vi "Math - Compute Impulse Response.vi"(0 "reference in":refnum<class "GSwFormDSP.lvclass">, 5 "error in (no error)":errorcluster) -> (14 "reference out":refnum<class "GSwFormDSP.lvclass">, 19 "error out":errorcluster)   [LabVIEW 2020, in "GSwFormDSP.lvclass"]
uses:
  GSwFormDSP.lvclass
  Attribute List.ctl
  Attribute Options.ctl
  <vilib>/Analysis/2dsp.llb/Inverse Real FFT.vi
  <vilib>/Analysis/NI_AALPro.lvlib
panel:
  out "Fs":dbl
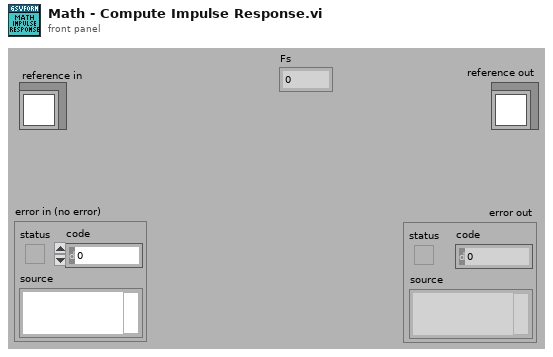
[diagram p1: front panel]
types:
  T1 = typedef "GSwFormDSP.lvclass/Attribute Options.ctl" = enum16{"Append to Attribute using \"( )\"", "Replace Attribute Value"}
  T2 = typedef "GSwFormDSP.lvclass/Attribute List.ctl" = string
  T3 = typedef "GSwFormDSP.lvclass/ObjectAttributes.ctl" = cluster{"Wform Ref":refnum<data-value>, "Nb Signals":i32, "Spectral Function Parameters":T4, "FFT":waveform(cdb)[], "Nb FFT":i32, "Nb Averages":i32[], "Reference Indexes":i32[], "Response Indexes":i32[], "Coherence":waveform(dbl)[], "TDF Parameters":T6, "DAQ":cluster{"Duration (sec)":dbl, "Buffer Size (Samples)":i32, "Offset (Samples)":i32}, "Filter Impulse Response (TDF)":waveform(dbl), "Sound Playback":T7}
  T4 = typedef "GSwFormDSP.lvclass/Spectral Parameters.ctl" = cluster{"Frequency resolution (Hz)":dbl, "Overlap":dbl, "Window":T5}
  T5 = typedef "NI_AALPro.lvlib/windowTd.ctl" = u32
  T6 = typedef "GSwFormDSP.lvclass/TDF Parameters.ctl" = cluster{"Filter":enum32{"Lowpass", "Highpass", "Bandpass", "Bandstop"}, "Type:":enum16{"Butterworth", "Chebyshev", "Inv Chebyshev", "Elliptic", "Bessel"}, "LP cutoff freq":dbl, "HP cutoff freq":dbl, "Order":i32, "passband ripple (dB)":dbl, "stopband attenuation (dB)":dbl, "Phaseless Filter":bool, "Include Fade IN and OUT":bool}
  T7 = typedef "GSwFormDSP.lvclass/Sound Playback.ctl" = cluster{"Timer start (ms)":u32, "task ID":T8, "Cursor Init Location (s)":dbl, "SC Volume":dbl}
  T8 = typedef "Sound Output Task ID.ctl" = u32
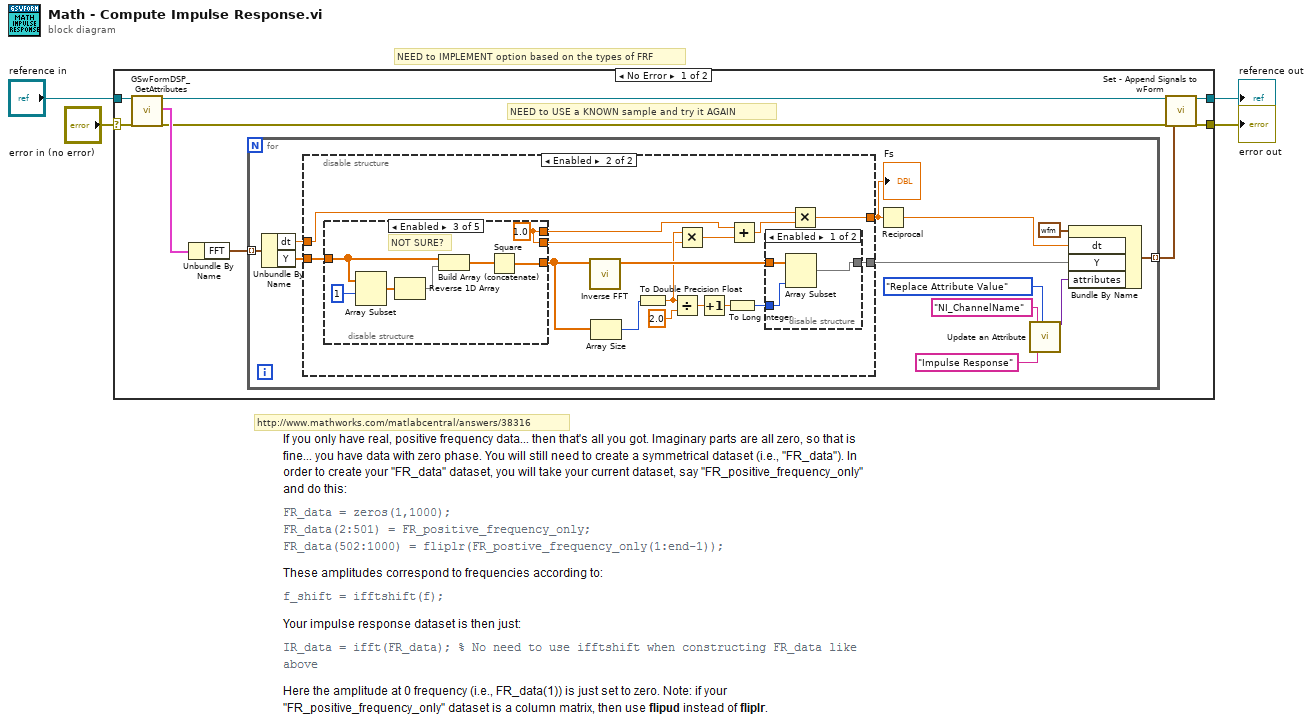
[diagram p0: block diagram]
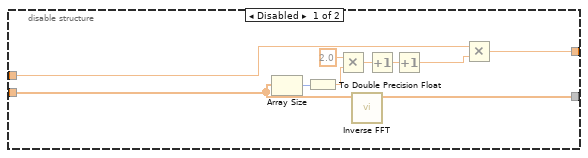
[diagram p2: hidden frame]
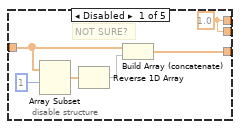
[diagram p4: hidden frame]
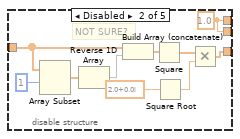
[diagram p5: hidden frame]
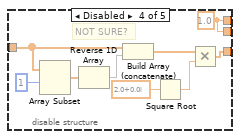
[diagram p6: hidden frame]
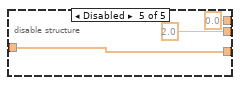
[diagram p7: hidden frame]
diagram:
  # "http://www.mathworks.com/matlabcentral/answers/38316"
  # "NEED to IMPLEMENT option based on the types of FRF"
  n1 = case shown="No Error" "error in (no error)" {
    selector: "error in (no error)" -> [w13 w92]
    tunnel: [w7 w92] -> w3
    tunnel: [w8 w91] -> w1
    tunnel: "reference in" -> [w12 w91]
    frame No Error {
      # "NEED to USE a KNOWN sample and try it AGAIN"
      n2 = call "GSwFormDSP_GetAttributes.vi"("reference in"=w12, "error in (no error)"=w13) -> ("reference out"=w9:refnum<class "GSwFormDSP.lvclass">, "attributes"=w11:T3, "error out"=w6:errorcluster)  [unwired: 14 in, 1 out]
      n3 = Unbundle By Name(w11) -> ("FFT"=w10:waveform(cdb)[])
      n4 = for {
        tunnel: w10 -> [w25] mode=indexing
        tunnel: [w21] -> w5 mode=indexing
        n5 = Unbundle By Name(w25) -> ("dt"=w19:dbl, "Y"=w20:cdb[])
        n6 = disable-structure shown="Enabled" {
          disable-tunnel: [w35 w36] -> w22
          disable-tunnel: w20 -> [w34 w44]
          disable-tunnel: w19 -> [w33 w51]
          disable-tunnel: [w31 w49] -> w18
          frame Disabled {
            n7 = Array Size(array=w34) -> (size(s)=w32:i32)
            n8 = To Double Precision Float(number=w32) -> (double precision float=w30:dbl)
            n9 = Multiply(x=2.0, y=w30) -> (x*y=w28:dbl)
            n10 = call-poly <vilib>:"Inverse FFT.vi"("FFT {X}"=w34) -> ("X"=w35:dbl[])  [unwired: 9 in, 1 out]
            n11 = Increment(x=w28) -> (x+1=w27:dbl)
            n12 = Increment(x=w27) -> (x+1=w26:dbl)
            n13 = Multiply(x=w33, y=w26) -> (x*y=w31:dbl)
          }
          frame Enabled {
            n14 = disable-structure shown="Enabled" {
              disable-tunnel: w44 -> [w58 w68 w75 w84 w90]
              disable-tunnel: [w56 w64 w72 w82 w90] -> w43
              disable-tunnel: [w59 w69 w76 w85 2.0 ("x")] -> w41
              disable-tunnel: [w59 w69 w76 w85 0.0 ("x")] -> w38
              frame Disabled {
                w59 = 1.0 ("x")
                # "NOT SURE?"
                n15 = Array Subset(array=w58, index=1) -> (w60:cdb[])  [unwired: 1 in]
                n16 = Reverse 1D Array(array=w60) -> (reversed array=w57:cdb[])
                n17 = Build Array (concatenate)(w58, w57) -> (w56:cdb[])
              }
              frame Disabled {
                w69 = 1.0 ("x")
                # "NOT SURE?"
                n18 = Array Subset(array=w68, index=1) -> (w70:cdb[])  [unwired: 1 in]
                n19 = Reverse 1D Array(array=w70) -> (reversed array=w67:cdb[])
                n20 = Build Array (concatenate)(w68, w67) -> (w66:cdb[])
                n21 = Square(x=w66) -> (x^2=w65:cdb[])
                n22 = Square Root(x=cdb 2.0+0.0i) -> (sqrt(x)=w63:cdb)
                n23 = Multiply(x=w65, y=w63) -> (x*y=w64:cdb[])
              }
              frame Enabled {
                w76 = 1.0 ("x")
                # "NOT SURE?"
                n24 = Array Subset(array=w75, index=1) -> (w77:cdb[])  [unwired: 1 in]
                n25 = Reverse 1D Array(array=w77) -> (reversed array=w74:cdb[])
                n26 = Build Array (concatenate)(w75, w74) -> (w73:cdb[])
                n27 = Square(x=w73) -> (x^2=w72:cdb[])
              }
              frame Disabled {
                w85 = 1.0 ("x")
                # "NOT SURE?"
                n28 = Array Subset(array=w84, index=1) -> (w86:cdb[])  [unwired: 1 in]
                n29 = Reverse 1D Array(array=w86) -> (reversed array=w83:cdb[])
                n30 = Build Array (concatenate)(w84, w83) -> (w79:cdb[])
                n31 = Square Root(x=cdb 2.0+0.0i) -> (sqrt(x)=w81:cdb)
                n32 = Multiply(x=w79, y=w81) -> (x*y=w82:cdb[])
              }
              frame Disabled {
              }
            }
            n33 = call-poly <vilib>:"Inverse FFT.vi"("FFT {X}"=w43) -> ("X"=w48:dbl[])  [unwired: 9 in, 1 out]
            n34 = Array Size(array=w43) -> (size(s)=w50:i32)
            n35 = To Double Precision Float(number=w50) -> (double precision float=w42:dbl)
            n36 = Divide(x=w42, y=2.0 ("x")) -> (x/y=w47:dbl)
            n37 = Multiply(x=w42, y=w41) -> (x*y=w40:dbl)
            n38 = Increment(x=w47) -> (x+1=w45:dbl)
            n39 = To Long Integer(number=w45) -> (32bit integer=w46:i32)
            n40 = Add(x=w38, y=w40) -> (x+y=w39:dbl)
            n41 = disable-structure shown="Enabled" {
              disable-tunnel: w48 -> [w54 w55]
              disable-tunnel: w46 -> [w53 _]
              disable-tunnel: [w52 w55] -> w36
              frame Enabled {
                n42 = Array Subset(array=w54, length=w53) -> (w52:dbl[])  [unwired: 1 in]
              }
              frame Disabled {
              }
            }
            n43 = Multiply(x=w51, y=w39) -> (x*y=w49:dbl)
          }
        }
        "Fs" <- w18
        n44 = Reciprocal(x=w18) -> (1/x=w24:dbl)
        n45 = call "Update an Attribute.vi"("Attribute List"=T2 "NI_ChannelName", "Attribute Value"="Impulse Response", "Attribute Option"=Attribute_Options."Replace Attribute Value") -> ("attributes out"=w16:variant)  [unwired: 15 in, 1 out]
        n46 = Bundle By Name(cluster=waveform(dbl) {"t0"=timestamp(0 s since 1904-01-01), "dt"=1.0, "Y"=[]} ("waveform"), "dt"=w24, "Y"=w22, "attributes"=w16) -> (w21:waveform(dbl))
      }
      n47 = call "Set - Append Signals to wForm.vi"("reference in"=w9, "error in (no error)"=w6, "New Signals"=w5) -> ("reference out"=w8:refnum<class "GSwFormDSP.lvclass">, "error out"=w7:errorcluster)  [unwired: 15 in]
    }
    frame Error {
    }
  }
  "error out" <- w3
  "reference out" <- w1
